vi "thermistor_param_init.vi"() -> ()   [LabVIEW 2018]
panel:
  out "Init Data Out":fxp<+,32,16>[](array[numeric])
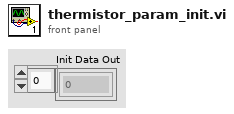
[diagram p1: front panel]
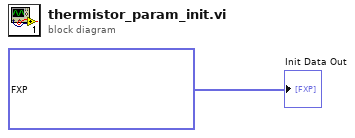
[diagram p0: block diagram]
diagram:
  "Init Data Out" <- fxp<+,32,16>[] [3434.0, 10.04779052734375, 3977.0, 62.06060791015625]
